vi "TestYPcopy.vi"() -> ()   [LabVIEW 2020, in "YP03-60CurrentSource_1.lvlib"]
uses:
  Libraries/YP03-60CurrentSource_1/YP03-60CurrentSource_1.lvlib
  <vilib>/Instr/_visa.llb/VISA Configure Serial Port (Instr).vi
panel:
  out "error out":errorcluster
  out "String":string
  out "return count 3":u32
  out "read buffer":string
  out "return count 2":u32
  out "String 2":string
  out "return count":u32
  out "Serial Settings:Number of Bytes at Serial Port":u32
  out "当前电流":string
  in  "error in (no error)":errorcluster
  in  "parity (0:none)":enum16{"None", "Odd", "Even", "Mark", "Space"}(ring)
  in  "data bits (8)":u16=8 min=5 max=8 step=1
  in  "baud rate (9600)":u32=9600
  in  "VISA resource name":refnum<visa-resource-name>
  out "输出控制":bool
  in  "电流设置":dbl min=-5.0 max=5.0 step=0.2
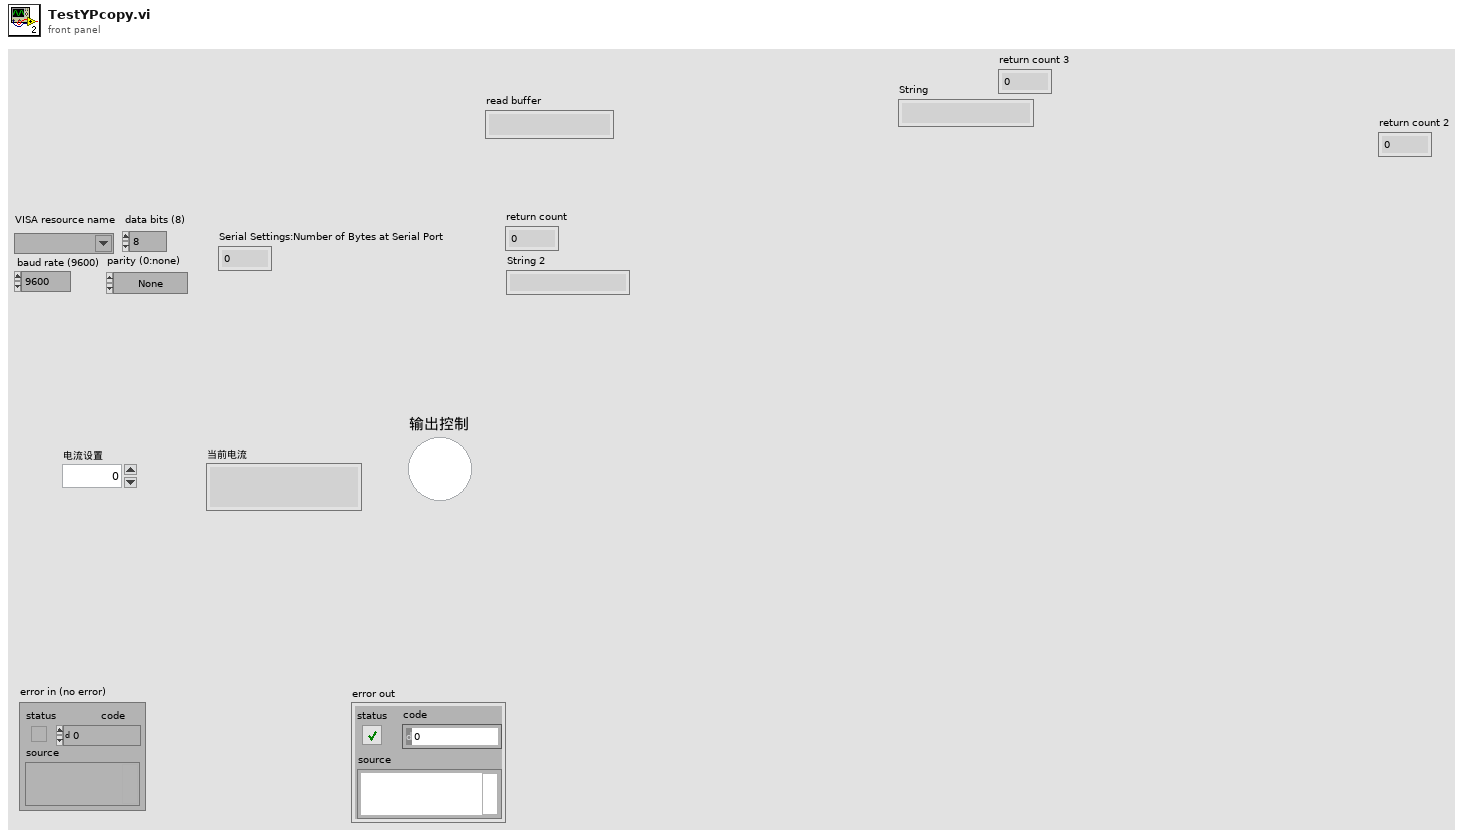
[diagram p1: front panel]
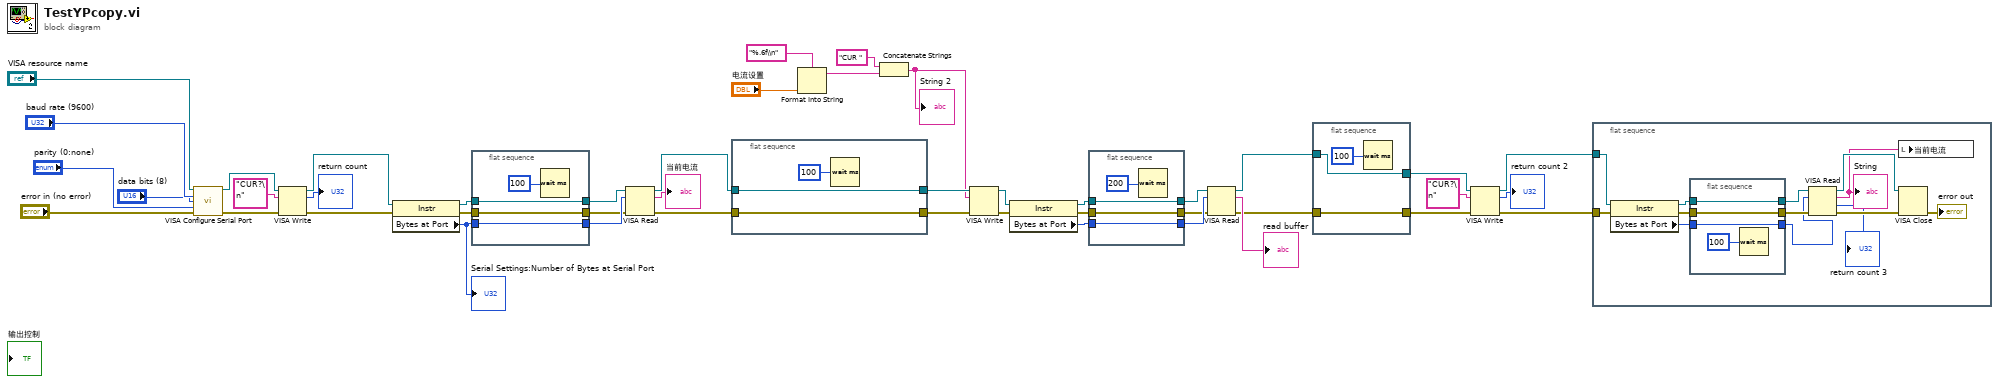
[diagram p0: block diagram]
diagram:
  n1 = call-poly "VISA Configure Serial Port"("VISA resource name"="VISA resource name", "baud rate (9600)"="baud rate (9600)", "data bits (8)"="data bits (8)", "parity (0:none)"="parity (0:none)", "error in (no error)"="error in (no error)") -> ("VISA resource name out"=w35:refnum<visa-resource-name>, "error out"=w34:errorcluster)  [unwired: 9 in]
  n2 = VISA Write(VISA resource name=w35, write buffer="CUR?\n", error in (no error)=w34) -> (VISA resource name out=w25:refnum<visa-resource-name>, return count=→"return count":u32, error out=w27:errorcluster)
  n3 = property class="Instr"(reference=w25, error in=w27) -> (reference out=w24:refnum<visa-resource-name>, error out=w26:errorcluster, "Bytes at Port"=w22:u32)
  "Serial Settings:Number of Bytes at Serial Port" <- w22
  n4 = flat-sequence {
    tunnel: w24 -> [w48]
    tunnel: [w48] -> w29
    tunnel: [w47] -> w1
    tunnel: w26 -> [w47]
    tunnel: [w46] -> w28
    tunnel: w22 -> [w46]
    frame #0 {
      n5 = Wait (ms)(milliseconds to wait=u32 100) -> ()  [unwired: 1 out]
    }
  }
  n6 = VISA Read(VISA resource name=w29, byte count=w28, error in (no error)=w1) -> (VISA resource name out=w21:refnum<visa-resource-name>, read buffer=→"当前电流":string, error out=w20:errorcluster)  [unwired: 1 out]
  n7 = flat-sequence {
    tunnel: w21 -> [w51]
    tunnel: [w51] -> w18
    tunnel: [w50] -> w19
    tunnel: w20 -> [w50]
    frame #0 {
      n8 = Wait (ms)(milliseconds to wait=u32 100) -> ()  [unwired: 1 out]
    }
  }
  n9 = Format Into String(format string="%.6f\\n", "电流设置") -> (resulting string=w41:string)  [unwired: 2 in, 1 out]
  n10 = Concatenate Strings("CUR " ("string"), w41) -> (w17:string)
  "String 2" <- w17
  n11 = VISA Write(VISA resource name=w18, write buffer=w17, error in (no error)=w19) -> (VISA resource name out=w31:refnum<visa-resource-name>, error out=w30:errorcluster)  [unwired: 1 out]
  n12 = property class="Instr"(reference=w31, error in=w30) -> (reference out=w7:refnum<visa-resource-name>, error out=w5:errorcluster, "Bytes at Port"=w9:u32)
  n13 = flat-sequence {
    tunnel: w7 -> [w55]
    tunnel: [w55] -> w6
    tunnel: [w54] -> w4
    tunnel: w5 -> [w54]
    tunnel: [w53] -> w8
    tunnel: w9 -> [w53]
    frame #0 {
      n14 = Wait (ms)(milliseconds to wait=u32 200) -> ()  [unwired: 1 out]
    }
  }
  n15 = VISA Read(VISA resource name=w6, byte count=w8, error in (no error)=w4) -> (VISA resource name out=w11:refnum<visa-resource-name>, read buffer=→"read buffer":string, error out=w3:errorcluster)  [unwired: 1 out]
  n16 = flat-sequence {
    tunnel: w11 -> [w58]
    tunnel: [w58] -> w12
    tunnel: [w56] -> w2
    tunnel: w3 -> [w56]
    frame #0 {
      n17 = Wait (ms)(milliseconds to wait=u32 100) -> ()  [unwired: 1 out]
    }
  }
  n18 = VISA Write(VISA resource name=w12, write buffer="CUR?\n", error in (no error)=w2) -> (VISA resource name out=w15:refnum<visa-resource-name>, return count=→"return count 2":u32, error out=w14:errorcluster)
  n19 = flat-sequence {
    tunnel: w15 -> [w68]
    tunnel: w14 -> [w66]
    frame #0 {
      n20 = property class="Instr"(reference=w68, error in=w66) -> (reference out=w69:refnum<visa-resource-name>, error out=w67:errorcluster, "Bytes at Port"=w70:u32)
      n21 = flat-sequence {
        tunnel: w69 -> [w75]
        tunnel: [w75] -> w65
        tunnel: [w74] -> w63
        tunnel: w67 -> [w74]
        tunnel: [w73] -> w59
        tunnel: w70 -> [w73]
        frame #0 {
          n22 = Wait (ms)(milliseconds to wait=u32 100) -> ()  [unwired: 1 out]
        }
      }
      n23 = VISA Read(VISA resource name=w65, byte count=w59, error in (no error)=w63) -> (VISA resource name out=w64:refnum<visa-resource-name>, read buffer=w61:string, return count=→"return count 3":u32, error out=w62:errorcluster)
      "String" <- w61
      n24 = local write "当前电流"(w61) -> ()
      n25 = VISA Close(VISA resource name=w64, error in (no error)=w62) -> (error out=→"error out":errorcluster)
    }
  }
